vi "Turn PID.vi"(8 "Range":dbl format="%#_13g", 11 "setpoint":dbl format="%.2f") -> (0 "in range?":bool, 2 "Right Out":dbl, 3 "Left Out":dbl)   [LabVIEW 2016]
uses:
  Robot Global Data.vi
  <vilib>/addons/control/pid/pid.llb/PID (DBL).vi
  <vilib>/addons/control/pid/NI_PID_pid.lvlib
panel:
  in  "minimum voltage":dbl=0.58 format="%#_13g"
  out "Yaw":dbl
  in  "PID gains":T1={"proportional gain (Kc)"=0.0225, "integral time (Ti, min)"=0.0, "derivative time (Td, min)"=0.0001}
  in  "output range":cluster{"output high":dbl, "output low":dbl}={"output high"=0.65, "output low"=-0.65}
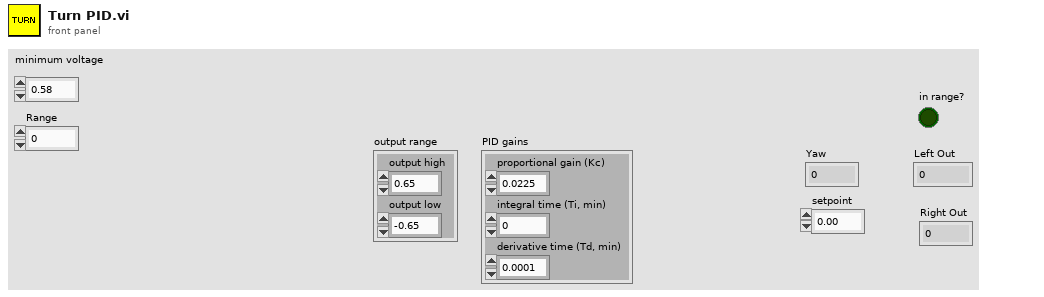
[diagram p1: front panel]
types:
  T1 = cluster{"proportional gain (Kc)":dbl, "integral time (Ti, min)":dbl, "derivative time (Td, min)":dbl}
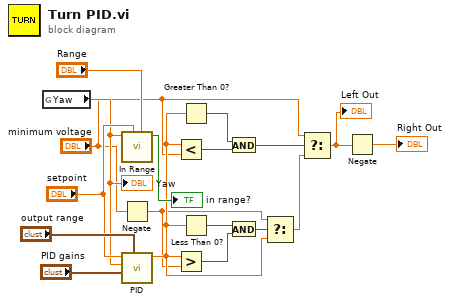
[diagram p0: block diagram]
diagram:
  n1 = global read "Robot Global Data.vi" "Yaw"() -> (w15:dbl)
  "Yaw" <- w15
  n2 = call "In Range.vi"("Range"="Range", "Setpoint"="setpoint", "Value"=w15) -> ("in range?"=→"in range?":bool)  [unwired: 8 in]
  n3 = Negate(x="minimum voltage") -> (-x=w1:dbl)
  n4 = call-poly <vilib>:"PID.vi"("output range"="output range", "PID gains"="PID gains", "process variable"=w15, "setpoint"="setpoint") -> ("output"=w5:dbl)  [unwired: 6 in, 1 out]
  n5 = Less?(x=w5, y="minimum voltage") -> (x < y?=w7:bool)
  n6 = Greater?(x=w5, y=w1) -> (0:w10:bool)
  n7 = Greater Than 0?(x=w5) -> (x > 0?=w6:bool)
  n8 = Less Than 0?(x=w5) -> (x < 0?=w11:bool)
  n9 = And(x=w6, y=w7) -> (x .and. y?=w8:bool)
  n10 = And(x=w11, y=w10) -> (x .and. y?=w9:bool)
  n11 = Select(t=w1, s=w9, f=w5) -> (s? t:f=w4:dbl)
  n12 = Select(t="minimum voltage", s=w8, f=w4) -> (s? t:f=w3:dbl)
  "Left Out" <- w3
  n13 = Negate(x=w3) -> (-x=→"Right Out":dbl)
